vi "Pointer producer consumer To Hexa Converter.vi"(10 "# Length":i32(ring) items=["U8", "U16", "U24", "U32", "U48", "U56", "U64"], 11 "NormalIn":string="\b\u0016$2HVd") -> (3 "Normal > Hex":string)   [LabVIEW 2014]
panel:
  # "Convert a Normal ASCII String   to  Hex String   with   Length"
  # "Tt"
  # "--"
  # "--"
  # "--"
  # "--"
  # "--"
  # "--"
  # "--"
  # "--"
  # "--"
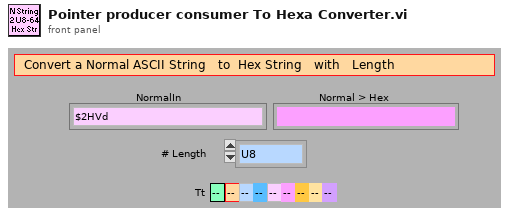
[diagram p1: front panel]
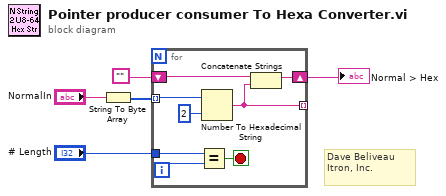
[diagram p0: block diagram]
diagram:
  # "Dave Beliveau\nItron, Inc."
  n1 = String To Byte Array(string="NormalIn") -> (unsigned byte array=w4:u8[])
  n2 = for {
    tunnel: w4 -> [w13] mode=indexing
    shift-right: [w11] -> w2
    shift-left: "" -> [w12]
    tunnel: [w10] -> _ mode=indexing
    tunnel: "# Length" -> [w7]
    i -> [w8]
    stop <- w6 stop-if-true
    n3 = Equal?(x=w7, y=w8) -> (x = y?=w6:bool)
    n4 = Number To Hexadecimal String(1:2, 2:w13) -> (0:w10:string)
    n5 = Concatenate Strings(w12, w10) -> (w11:string)
  }
  "Normal > Hex" <- w2
